vi "available tag dialog.vi"(7 "channel action event":refnum<user-event>, 8 "error in":errorcluster, 10 "channel to map to":refnum<class "TBM channel.lvclass">, 11 "filtered tags":refnum<class "tag descriptor.lvclass">[](array[class])) -> (0 "error out":errorcluster)   [LabVIEW 2013, in "Table Manager.lvlib"]
uses:
  Table Manager.lvlib
  <vilib>/NI/Tag Bus/tag/tag descriptor.lvclass
  channel action event.ctl
  dialog output action.ctl
  <vilib>/NI/Tag Bus Module Framework/channel/TBM channel.lvclass
  Table Manager/Call Back Ref Type Def.ctl
  Configuration Editor/Classes/Engine Parent/Engine Parent Editor Node.lvclass
  Configuration Editor/Classes/Module editor node/module editor node.lvclass
  <vilib>/event_ctls.llb/usereventprio.ctl
  <vilib>/NI/Tag Bus/tag/tag descriptor.lvclass/tag descriptor.ctl
  Table Manager/Table Manager.lvclass
panel:
  in  "Set Default":bool
  in  "Create Tag":bool
  in  "Filter":string
  in  "Available Tags":i32(listbox)
  in  "disconnect":bool
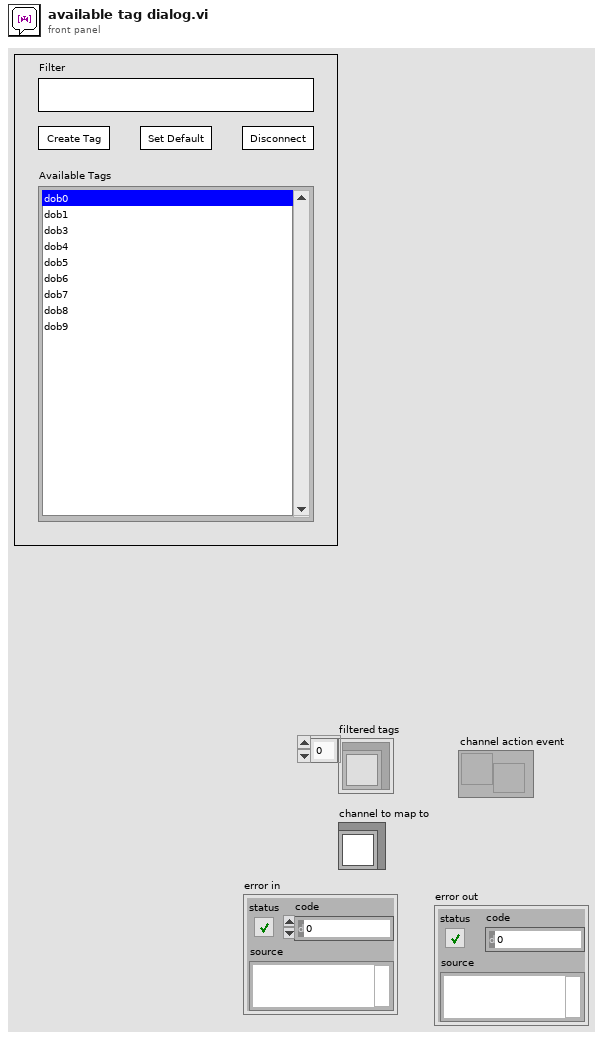
[diagram p1: front panel]
types:
  T1 = typedef "usereventprio.ctl" = enum32{"high priority", "normal priority"}
  T2 = typedef "Table Manager.lvlib/dialog output action.ctl" = enum16{"Tag Created", "Tag Selected", "Set Default", "disconnect"}
  T3 = typedef "Table Manager.lvlib/channel action event.ctl" = cluster{"action":T2, "channel":refnum<class "TBM channel.lvclass">, "selected tag":refnum<class "tag descriptor.lvclass">, "Call Back VI":T4}
  T4 = typedef "Table Manager.lvlib/Table Manager.lvclass/Call Back Ref Type Def.ctl" = refnum<vi>
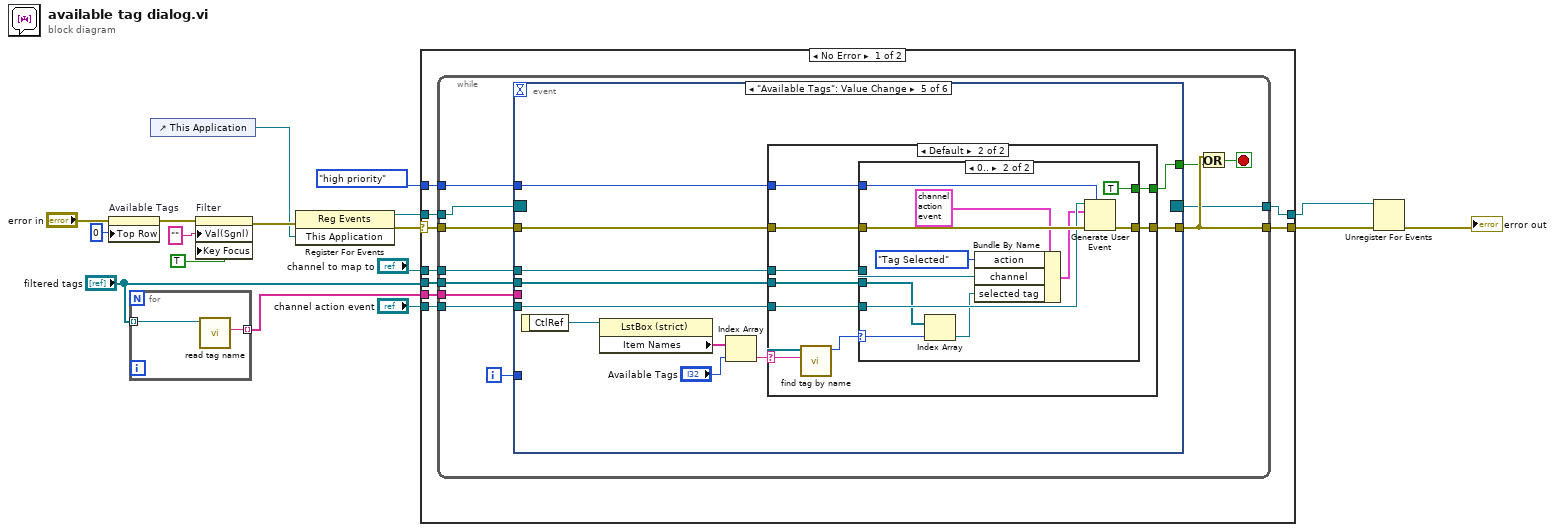
[diagram p0: block diagram]
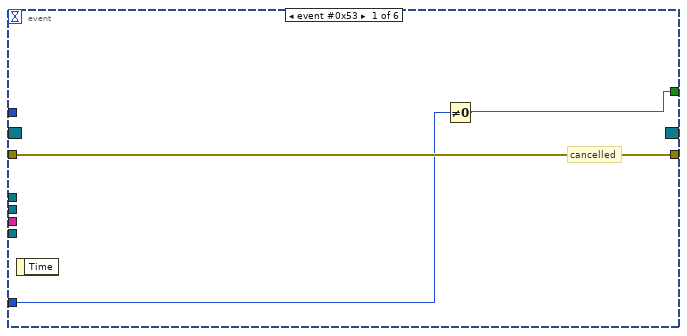
[diagram p2: hidden frame]
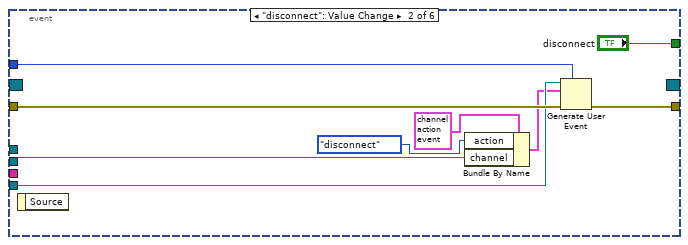
[diagram p3: hidden frame]
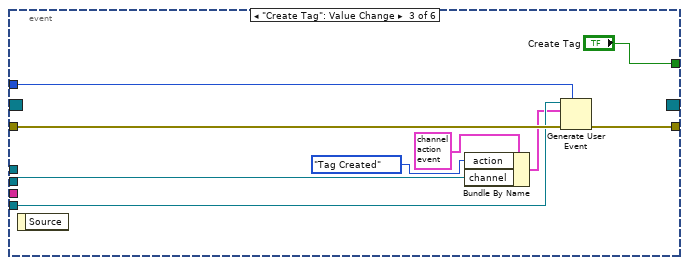
[diagram p4: hidden frame]
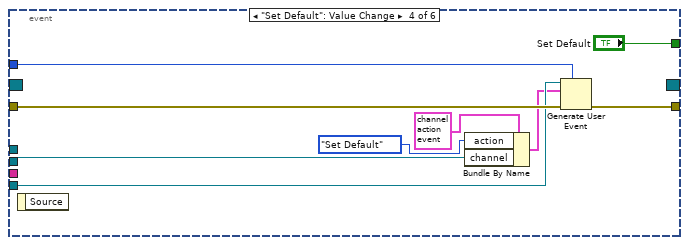
[diagram p5: hidden frame]
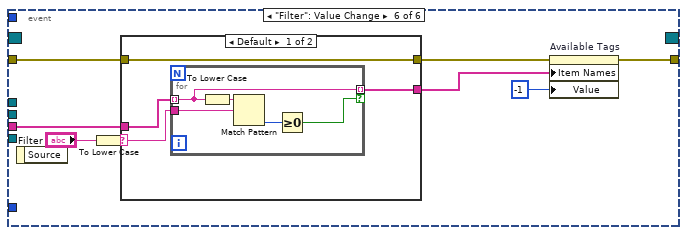
[diagram p8: hidden frame]
diagram:
  n1 = property on="Available Tags" class="LstBox (strict)"(error in="error in", "Top Row"=0) -> (error out=w1:errorcluster)  [unwired: 1 in, 1 out]
  n2 = for {
    tunnel: "filtered tags" -> [w19] mode=indexing
    tunnel: [w18] -> w12 mode=indexing
    n3 = call <vilib>:"read tag name.vi"("system tag in"=w19) -> ("name"=w18:string)  [unwired: 8 in, 2 out]
  }
  n4 = control-ref of="This Application"() -> (w4:refnum<vi>)
  n5 = property on="Filter" class="Str"(error in=w1, "Val(Sgnl)"="" ("Value (Signaling)"), "Key Focus"=TRUE) -> (error out=w11:errorcluster)  [unwired: 1 in, 1 out]
  n6 = register-events(error in=w11, w4) -> (reference out=w7:refnum<event-registration>, error out=w8:errorcluster)  [unwired: 1 in]
  n7 = case shown="No Error" w8 {
    selector: w8 -> [w26 w125]
    tunnel: [w28 w125] -> w17
    tunnel: "channel action event" -> [w27 _]
    tunnel: "channel to map to" -> [w25 _]
    tunnel: usereventprio."high priority" ("priority (normal)") -> [w24 _]
    tunnel: "filtered tags" -> [w23 _]
    tunnel: w12 -> [w22 _]
    tunnel: w7 -> [w21 w124]
    tunnel: [w20 w124] -> w5
    frame No Error {
      n8 = while {
        tunnel: w26 -> [w40]
        tunnel: [w38] -> w28
        tunnel: w27 -> [w36]
        tunnel: w25 -> [w35]
        tunnel: w24 -> [w34]
        tunnel: w23 -> [w33]
        tunnel: w22 -> [w32]
        tunnel: w21 -> [w30]
        tunnel: [w29] -> w20
        i -> [w31]
        stop <- w39 stop-if-true
        n9 = event shown="[4] \"Available Tags\": Value Change" {
          selector: w30 -> [_ _ _ _ _ _]
          dyn-events: [_ _ _ _ _ _] -> w29
          timeout: _ -> [_ _ _ _ _ _]
          tunnel: w40 -> [w43 w52 w61 w70 w81 w112]
          tunnel: [w43 w51 w60 w69 w80 w109] -> w38
          tunnel: [w42 "disconnect" "Create Tag" "Set Default" w72 _] -> w37
          tunnel: w36 -> [_ w50 w59 w68 w79 _]
          tunnel: w35 -> [_ w46 w55 w64 w78 _]
          tunnel: w34 -> [_ w45 w54 w63 w77 _]
          tunnel: w33 -> [_ _ _ _ w73 _]
          tunnel: w32 -> [_ _ _ _ _ w106]
          tunnel: w31 -> [w41 _ _ _ _ _]
          event event #0x53 {
            # "cancelled"
            n10 = event-data() -> ()  [unwired: 1 in, 1 out]
            n11 = Not Equal To 0?(x=w41) -> (x != 0?=w42:bool)
          }
          event "disconnect": Value Change {
            n12 = event-data() -> ()  [unwired: 1 in, 1 out]
            n13 = Bundle By Name(cluster=T3 {"action"=enum."Tag Created", "channel"=refnum, "selected tag"=refnum, "Call Back VI"=refnum} ("event data"), "action"=dialog_output_action."disconnect", "channel"=w46) -> (w48:T3)
            n14 = Generate User Event(priority (normal)=w45, user event=w50, event data cluster=w48, error in=w52) -> (error out=w51:errorcluster)  [unwired: 1 out]
          }
          event "Create Tag": Value Change {
            n15 = event-data() -> ()  [unwired: 1 in, 1 out]
            n16 = Bundle By Name(cluster=T3 {"action"=enum."Tag Created", "channel"=refnum, "selected tag"=refnum, "Call Back VI"=refnum} ("event data"), "action"=dialog_output_action."Tag Created", "channel"=w55) -> (w57:T3)
            n17 = Generate User Event(priority (normal)=w54, user event=w59, event data cluster=w57, error in=w61) -> (error out=w60:errorcluster)  [unwired: 1 out]
          }
          event "Set Default": Value Change {
            n18 = event-data() -> ()  [unwired: 1 in, 1 out]
            n19 = Bundle By Name(cluster=T3 {"action"=enum."Tag Created", "channel"=refnum, "selected tag"=refnum, "Call Back VI"=refnum} ("event data"), "action"=dialog_output_action."Set Default", "channel"=w64) -> (w66:T3)
            n20 = Generate User Event(priority (normal)=w63, user event=w68, event data cluster=w66, error in=w70) -> (error out=w69:errorcluster)  [unwired: 1 out]
          }
          event "Available Tags": Value Change {
            n21 = event-data() -> ("CtlRef"=w76:refnum<vi>)  [unwired: 1 in]
            n22 = property class="LstBox (strict)"(reference=w76) -> ("Item Names"=w75:string[])  [unwired: 1 in, 2 out]
            n23 = Index Array(array=w75, index="Available Tags") -> (element=w74:string)
            n24 = case shown="Default" w74 {
              selector: w74 -> [_ w86]
              tunnel: w81 -> [w82 w91]
              tunnel: [w82 w90] -> w80
              tunnel: w79 -> [_ w89]
              tunnel: w78 -> [_ w88]
              tunnel: w77 -> [_ w87]
              tunnel: w73 -> [_ w84]
              tunnel: [_ w83] -> w72
              frame "" {
              }
              frame Default {
                n25 = call <vilib>:"find tag by name.vi"("name"=w86, "tags in"=w84) -> ("index"=w85:i32)  [unwired: 9 in]
                n26 = case shown="0.." w85 {
                  selector: w85 -> [_ w96]
                  tunnel: w91 -> [w92 w104]
                  tunnel: [w92 w103] -> w90
                  tunnel: w89 -> [_ w102]
                  tunnel: w88 -> [_ w98]
                  tunnel: w87 -> [_ w97]
                  tunnel: w84 -> [_ w95]
                  tunnel: [_ TRUE] -> w83
                  frame ..-1 {
                  }
                  frame 0.. {
                    n27 = Index Array(array=w95, index=w96) -> (element=w94:refnum<class "tag descriptor.lvclass">)
                    n28 = Bundle By Name(cluster=T3 {"action"=enum."Tag Created", "channel"=refnum, "selected tag"=refnum, "Call Back VI"=refnum} ("event data"), "action"=dialog_output_action."Tag Selected", "channel"=w98, "selected tag"=w94) -> (w100:T3)
                    n29 = Generate User Event(priority (normal)=w97, user event=w102, event data cluster=w100, error in=w104) -> (error out=w103:errorcluster)  [unwired: 1 out]
                  }
                }
              }
            }
          }
          event "Filter": Value Change {
            n30 = event-data() -> ()  [unwired: 1 in, 1 out]
            n31 = To Lower Case(string="Filter") -> (all lower case string=w105:string)
            n32 = case shown="Default" w105 {
              selector: w105 -> [w115 _]
              tunnel: w112 -> [w116 w123]
              tunnel: [w116 w123] -> w108
              tunnel: [w113 w122] -> w107
              tunnel: w106 -> [w114 w122]
              frame Default {
                n33 = for {
                  tunnel: w115 -> [w121]
                  tunnel: w114 -> [w120] mode=indexing
                  tunnel: [w120] -> w113 mode=indexing if=w118
                  n34 = To Lower Case(string=w120) -> (all lower case string=w117:string)
                  n35 = Match Pattern(string=w117, regular expression=w121) -> (offset past match=w119:i32)  [unwired: 1 in, 3 out]
                  n36 = Greater Or Equal To 0?(x=w119) -> (x >= 0?=w118:bool)
                }
              }
              frame "" {
              }
            }
            n37 = property on="Available Tags" class="LstBox (strict)"(error in=w108, "Item Names"=w107, "Value"=-1 ("Available Tags")) -> (error out=w109:errorcluster)  [unwired: 1 in, 1 out]
          }
        }
        n38 = Or(x=w38, y=w37) -> (x .or. y?=w39:bool)
      }
    }
    frame Error {
    }
  }
  n39 = Unregister For Events(event registration refnum=w5, error in=w17) -> (error out=→"error out":errorcluster)
